vi "Configure Control Parameters.vi"(0 "VISA resource name":refnum<visa-resource-name>, 1 "Gain (P) (0.0)":dbl format="%.1f", 2 "Reset (I) (0.0)":dbl format="%.1f", 3 "Rate (D) (0 %)":u16, 5 "Loop (1:Loop 1)":u16(ring)=1 items=["Loop 1"=1, "Loop 2"=2], 7 "Heater Range (0:Off)":u16(ring) items=["Off", "Low (loop 1) or On (loop 2)", "High (loop 1)"], 9 "Heater Resistance (1:25 Ohm)":u16(ring)=1 items=["25 Ohm"=1, "50 Ohm"=2], 11 "error in (no error)":errorcluster, 12 "Manual Heater Power (0.000 %)":dbl format="%.3f") -> (4 "VISA resource name out":refnum<visa-resource-name>, 15 "error out":errorcluster)   [LabVIEW 2019, in "Lake Shore 325.lvlib"]
doc: "This vi configures control parameters - PID, Manual Heater Output, Heater Range, and Heater Resistance."
uses:
  Lake Shore 325.lvlib
  Instance           1 36Saved   Configure Control Parameters .vi
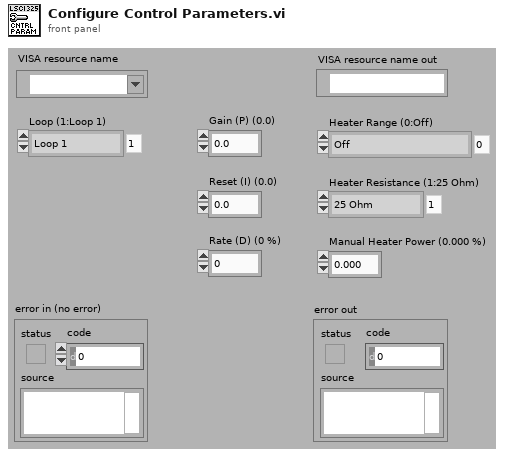
[diagram p1: front panel]
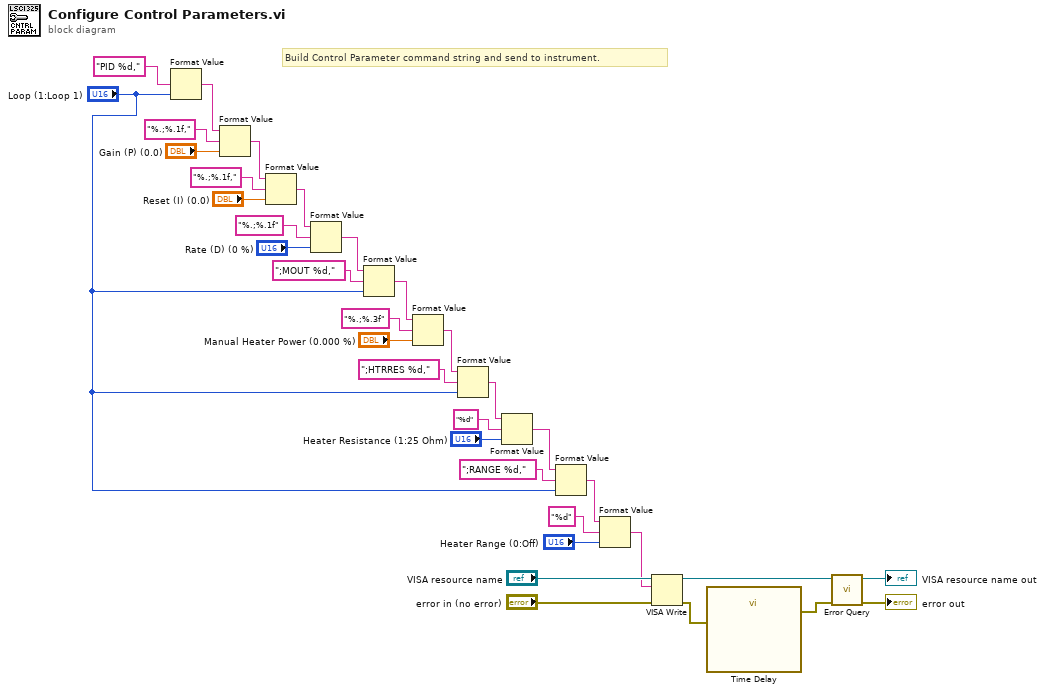
[diagram p0: block diagram]
diagram:
  # "Build Control Parameter command string and send to instrument."
  n1 = Format Value(format string="PID %d,", value (0)="Loop (1:Loop 1)") -> (output string=w10:string)  [unwired: 1 in]
  n2 = Format Value(string ("")=w10, format string="%.;%.1f,", value (0)="Gain (P) (0.0)") -> (output string=w24:string)
  n3 = Format Value(string ("")=w24, format string="%.;%.1f,", value (0)="Reset (I) (0.0)") -> (output string=w21:string)
  n4 = Format Value(string ("")=w21, format string="%.;%.1f", value (0)="Rate (D) (0 %)") -> (output string=w9:string)
  n5 = Format Value(string ("")=w9, format string=";MOUT %d,", value (0)="Loop (1:Loop 1)") -> (output string=w8:string)
  n6 = Format Value(string ("")=w8, format string="%.;%.3f", value (0)="Manual Heater Power (0.000 %)") -> (output string=w7:string)
  n7 = Format Value(string ("")=w7, format string=";HTRRES %d,", value (0)="Loop (1:Loop 1)") -> (output string=w6:string)
  n8 = Format Value(string ("")=w6, format string="%d", value (0)="Heater Resistance (1:25 Ohm)") -> (output string=w5:string)
  n9 = Format Value(string ("")=w5, format string=";RANGE %d,", value (0)="Loop (1:Loop 1)") -> (output string=w4:string)
  n10 = Format Value(string ("")=w4, format string="%d", value (0)="Heater Range (0:Off)") -> (output string=w31:string)
  n11 = VISA Write(VISA resource name="VISA resource name", write buffer=w31, error in (no error)="error in (no error)") -> (VISA resource name out=w30:refnum<visa-resource-name>, error out=w2:errorcluster)  [unwired: 1 out]
  n12 = call "Time Delay"("error in (no error)"=w2) -> ("error out"=w1:errorcluster)  [unwired: 10 in]
  n13 = call "Error Query.vi"("error in (no error)"=w1, "VISA resource name"=w30) -> ("error out"=→"error out":errorcluster, "VISA resource name out"=→"VISA resource name out":refnum<visa-resource-name>)  [unwired: 7 in, 1 out]
